vi "PID.vi"(0 "Des theta0":dbl, 1 "PID gains":T1={"proportional gain (Kc)"=1.0, "integral time (Ti, min)"=0.01, "derivative time (Td, min)"=0.0} {"derivative time (Td, min)" format="%.3f"; "integral time (Ti, min)" format="%.3f"; "proportional gain (Kc)" format="%.3f"}, 2 "NewTarget":bool, 5 "Des theta1":dbl, 7 "current theta0":dbl, 9 "current theta1":dbl, 11 "error in (no error)":errorcluster) -> (4 "U1":dbl, 6 "U2":dbl, 8 "Dir1":bool, 10 "Dir2":bool, 15 "error out":errorcluster)   [LabVIEW 2017, in "admittanceControllerLibrary.lvlib"]
uses:
  admittanceControllerLibrary.lvlib
  <vilib>/addons/control/pid/pid.llb/PID (DBL).vi
  <vilib>/addons/control/pid/NI_PID_pid.lvlib
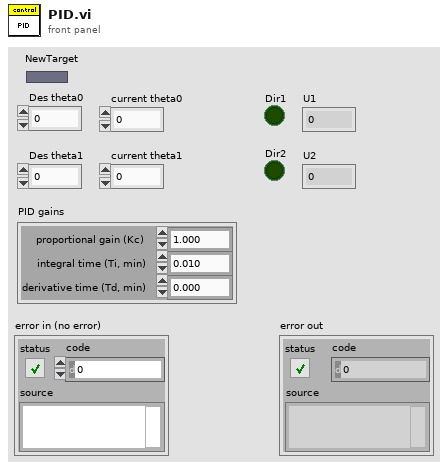
[diagram p1: front panel]
types:
  T1 = cluster{"proportional gain (Kc)":dbl, "integral time (Ti, min)":dbl, "derivative time (Td, min)":dbl}
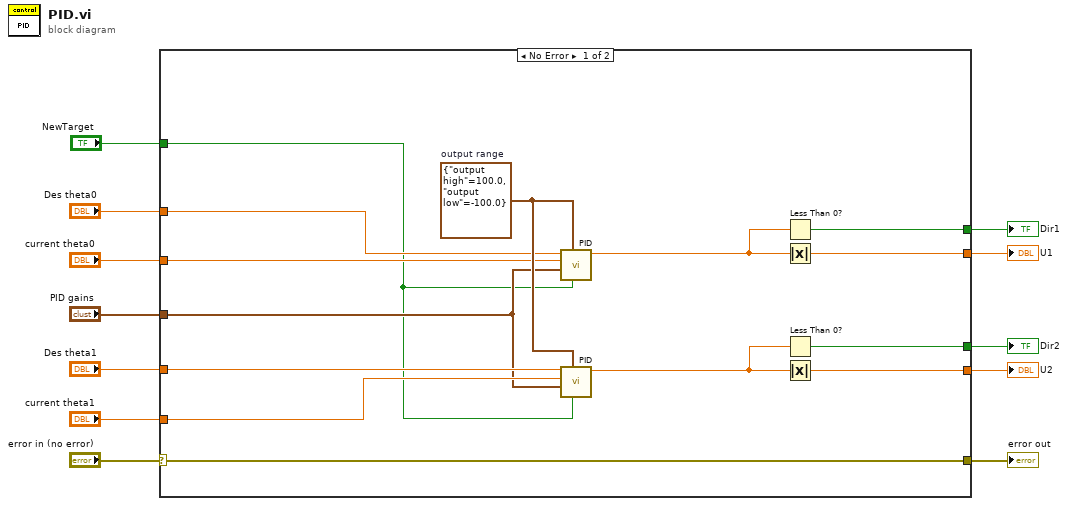
[diagram p0: block diagram]
diagram:
  n1 = case shown="No Error" "error in (no error)" {
    selector: "error in (no error)" -> [w23 w27]
    tunnel: [w23 w27] -> w11
    tunnel: "current theta1" -> [w22 _]
    tunnel: "current theta0" -> [w21 _]
    tunnel: "Des theta0" -> [w20 _]
    tunnel: "Des theta1" -> [w19 _]
    tunnel: "PID gains" -> [w18 _]
    tunnel: [w17 _] -> w5
    tunnel: [w16 _] -> w4
    tunnel: [w15 _] -> w3
    tunnel: [w14 _] -> w2
    tunnel: "NewTarget" -> [w13 _]
    frame No Error {
      w26 = cluster{"output high":dbl, "output low":dbl} {"output high"=100.0, "output low"=-100.0}  # output range
      n2 = call-poly <vilib>:"PID.vi"("reinitialize? (F)"=w13, "output range"=w26, "PID gains"=w18, "process variable"=w21, "setpoint"=w20) -> ("output"=w25:dbl)  [unwired: 5 in, 1 out]
      n3 = call-poly <vilib>:"PID.vi"("reinitialize? (F)"=w13, "output range"=w26, "PID gains"=w18, "process variable"=w22, "setpoint"=w19) -> ("output"=w24:dbl)  [unwired: 5 in, 1 out]
      n4 = Less Than 0?(x=w25) -> (x < 0?=w16:bool)
      n5 = Absolute Value(x=w25) -> (abs(x)=w14:dbl)
      n6 = Less Than 0?(x=w24) -> (x < 0?=w17:bool)
      n7 = Absolute Value(x=w24) -> (abs(x)=w15:dbl)
    }
    frame Error {
    }
  }
  "error out" <- w11
  "U1" <- w2
  "U2" <- w3
  "Dir1" <- w4
  "Dir2" <- w5
